vi "TARGET.vi"() -> ()   [LabVIEW 2015]
panel:
  in  "Table":string[][](table)
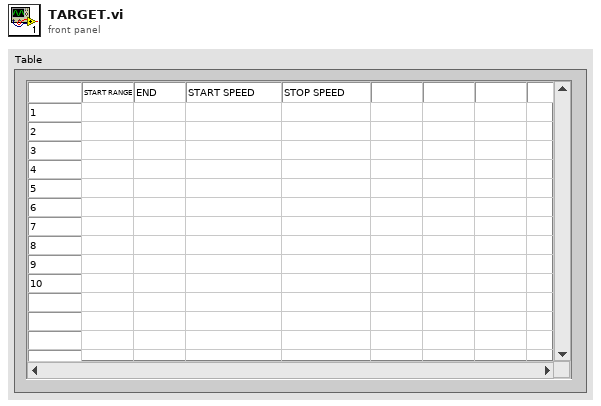
[diagram p1: front panel]
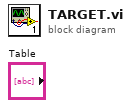
[diagram p0: block diagram]
diagram:
